vi "Read hSysLog.vi"(8 "error in":errorcluster, 11 "Text Device Session in":refnum<class "Text Device Session.lvclass">) -> (0 "error out":errorcluster, 2 "Session Handle":T1, 3 "Text Device Session out":refnum<class "Text Device Session.lvclass">)   [LabVIEW 2018, in "Text Device Session.lvclass"]
uses:
  Text Device Session.lvclass
  <vilib>/MSR Consulting, LLC/General Reuse/Session APIs/_Session Fwk/Typedefs/Session Handle.ctl
  <vilib>/MSR Consulting, LLC/General Reuse/Session APIs/_Session Fwk/Session - Root.lvclass
  Text Device Session.lvclass/Text Device Session.ctl
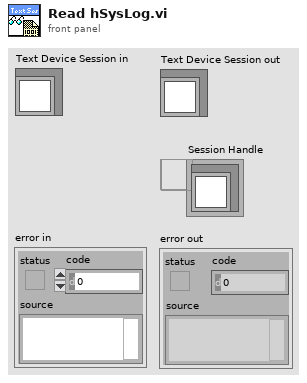
[diagram p1: front panel]
types:
  T1 = typedef "Session - Root.lvclass/Session Handle.ctl" = refnum<data-value>
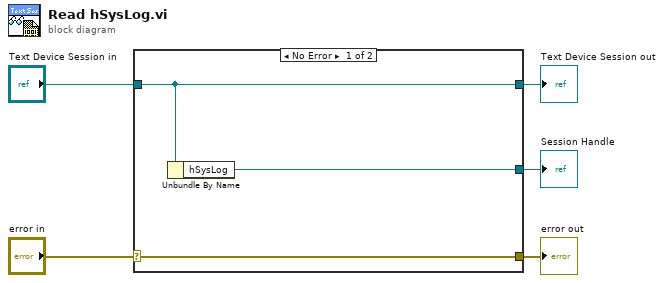
[diagram p0: block diagram]
diagram:
  n1 = case shown="No Error" "error in" {
    selector: "error in" -> [w8 w9]
    tunnel: [w8 w9] -> w4
    tunnel: [w7 w10] -> w2
    tunnel: "Text Device Session in" -> [w7 w10]
    tunnel: [w6 _] -> w1
    frame No Error {
      n2 = Unbundle By Name(w7) -> ("hSysLog"=w6:T1)
    }
    frame Error {
    }
  }
  "error out" <- w4
  "Text Device Session out" <- w2
  "Session Handle" <- w1
